vi "OpenVeriStandConnection.vi"(6 "Gateway IP Address (\"\": localhost)":string, 8 "error in (no error)":errorcluster, 9 "overrides files":path[](array[path]), 10 "System Definition File":path, 11 "VeriStand Test Case in":refnum<class "VeriStandTestCase.lvclass">) -> (0 "error out":errorcluster, 3 "VeriStand Test Case out":refnum<class "VeriStandTestCase.lvclass">)   [LabVIEW 2015, in "VeriStandTestCase.lvclass"]
uses:
  VeriStandTestCase.lvclass
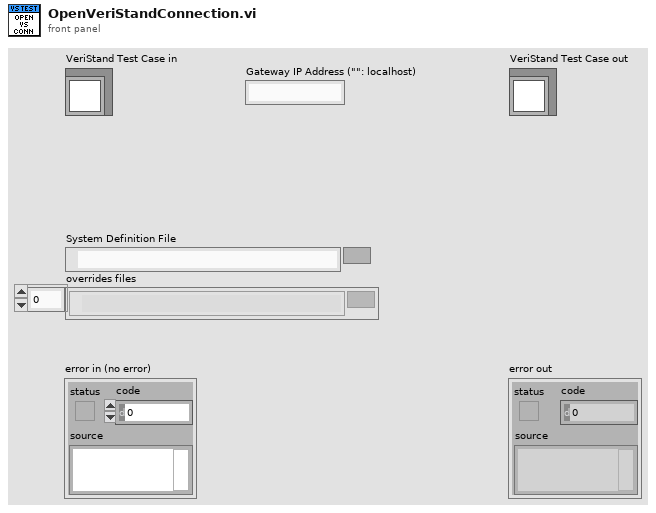
[diagram p1: front panel]
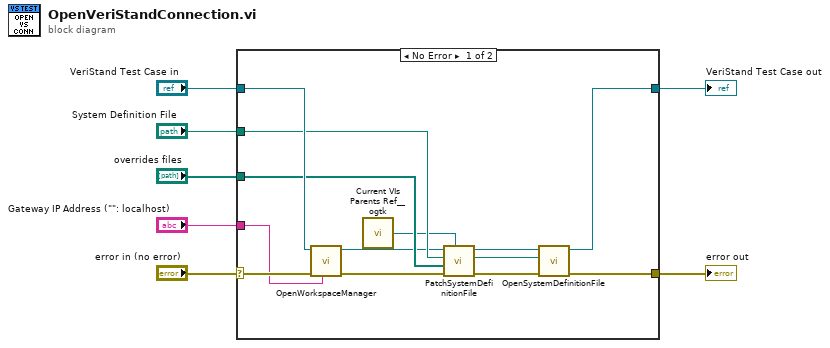
[diagram p0: block diagram]
diagram:
  n1 = case shown="No Error" "error in (no error)" {
    selector: "error in (no error)" -> [w18 w22]
    tunnel: [w19 w22] -> w6
    tunnel: [w20 w21] -> w4
    tunnel: "VeriStand Test Case in" -> [w17 w21]
    tunnel: "System Definition File" -> [w14 _]
    tunnel: "Gateway IP Address (\"\": localhost)" -> [w16 _]
    tunnel: "overrides files" -> [w13 _]
    frame No Error {
      n2 = call "OpenWorkspaceManager.vi"("Gateway IP Address (\"\": localhost)"=w16, "error in (no error)"=w18, "VeriStandTestCase in"=w17) -> ("error out"=w15:errorcluster, "VeriStandTestCase out"=w8:refnum<class "VeriStandTestCase.lvclass">)  [unwired: 7 in]
      n3 = call <userlib>:"Current VIs Parents Ref__ogtk.vi"() -> ("Calling VI's Reference"=w9:refnum<vi>)  [unwired: 2 in]
      n4 = call "PatchSystemDefinitionFile.vi"("VI in"=w9, "error in (no error)"=w15, "overrides files"=w13, "System Definition File"=w14, "VeriStand Test Case in"=w8) -> ("error out"=w12:errorcluster, "absolute overridden system definition file"=w10:path, "VeriStand Test Case out"=w11:refnum<class "VeriStandTestCase.lvclass">)  [unwired: 4 in]
      n5 = call "OpenSystemDefinitionFile.vi"("error in (no error)"=w12, "absolute system definition file"=w10, "VeriStand Test Case in"=w11) -> ("error out"=w19:errorcluster, "VeriStand Test Case out"=w20:refnum<class "VeriStandTestCase.lvclass">)  [unwired: 7 in]
    }
    frame Error {
    }
  }
  "error out" <- w6
  "VeriStand Test Case out" <- w4
